vi "factory Reset.vi"(7 "option":u8, 9 "id":u8, 10 "protocol_version":i32, 11 "port_num":i32) -> ()   [LabVIEW 2015, in "dxl_x86_c.lvlib"]
doc: "WINDECLSPEC void factoryReset (int port_num, int protocol_version, uint8_t id, uint8_t option);"
uses:
  dxl_x86_c.lvlib
  dxl_x86_c.dll
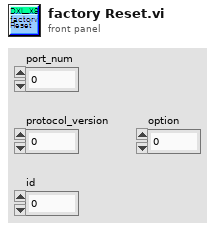
[diagram p1: front panel]
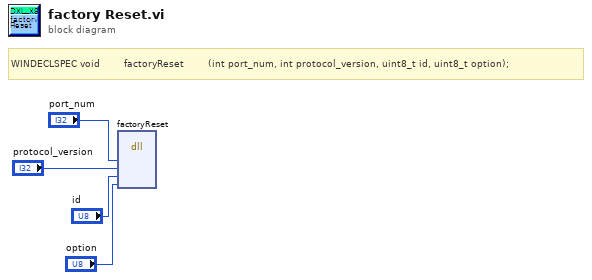
[diagram p0: block diagram]
diagram:
  # "WINDECLSPEC void        factoryReset        (int port_num, int protocol_version, uint8_t id, uint8_t option);"
  n1 = dll-call lib="C:/Users/Platform/Desktop/LabVIEW/dxl_x86_c.lvlib/dxl_x86_c.*" fn="factoryReset"("port_num"="port_num", "protocol_version"="protocol_version", "id"="id", "option"="option") -> ()  [unwired: 8 in, 2 out]
